vi "InitFromXML.vi"(8 "error in (no error)":errorcluster, 10 "XML":string, 11 "RingItemProjectWizard in":refnum<class "RingItemProjectWizard.lvclass">) -> (0 "error out":errorcluster, 3 "RingItemProjectWizard out":refnum<class "RingItemProjectWizard.lvclass">)   [LabVIEW 2009, in "NavScreen.lvlib" / "RingItemProjectWizard.lvclass"]
uses:
  RingItemProjectWizard.lvclass
  RingItem/RingItem.lvclass
  RingItemProjectWizard.lvclass/RingItemProjectWizard.ctl
  NavScreen.lvlib
  ProjectWizard/ProjectWizard.lvclass
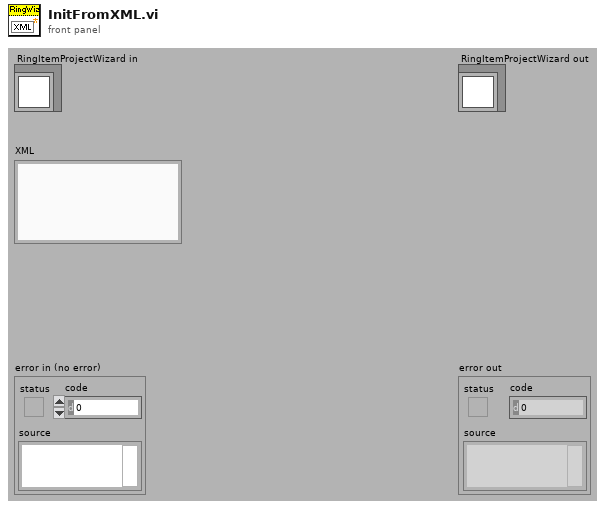
[diagram p1: front panel]
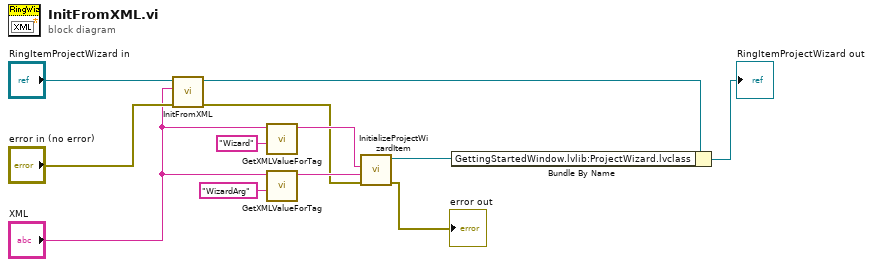
[diagram p0: block diagram]
diagram:
  n1 = call-parent "InitFromXML.vi"("error in (no error)"="error in (no error)", "XML"="XML", "RingItem in"="RingItemProjectWizard in") -> ("error out"=w3:errorcluster, "RingItem out"=w6:refnum<class "RingItemProjectWizard.lvclass">)  [unwired: 7 in]
  n2 = call "GetXMLValueForTag.vi"("tag"="Wizard", "XML"="XML") -> ("value"=w8:string)  [unwired: 8 in, 1 out]
  n3 = call "GetXMLValueForTag.vi"("tag"="WizardArg", "XML"="XML") -> ("value"=w7:string)  [unwired: 8 in, 1 out]
  n4 = call "InitializeProjectWizardItem.vi"("error in (no error)"=w3, "wizard argument"=w7, "wizard"=w8) -> ("error out"=→"error out":errorcluster, "ProjectWizard out"=w5:refnum<class "ProjectWizard.lvclass">)  [unwired: 7 in]
  n5 = Bundle By Name(cluster=w6, "GettingStartedWindow.lvlib:ProjectWizard.lvclass"=w5) -> (→"RingItemProjectWizard out":refnum<class "RingItemProjectWizard.lvclass">)
